vi "Get StartStop Status.vi"(8 "error in":errorcluster, 11 "VISA resource name in":refnum<visa-resource-name>) -> (0 "error out":errorcluster, 1 "Status":bool, 3 "VISA resource name out":refnum<visa-resource-name>)   [LabVIEW 2015, in "JULABO DeviceDriver.lvlib"]
doc: "This VI returns true if the instrument is started or false if it is in Standby-Mode"
uses:
  JULABO DeviceDriver.lvlib
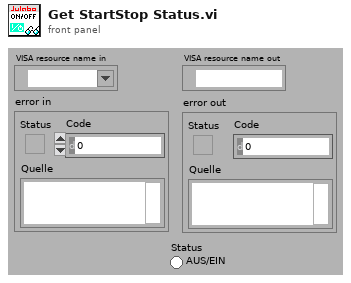
[diagram p1: front panel]
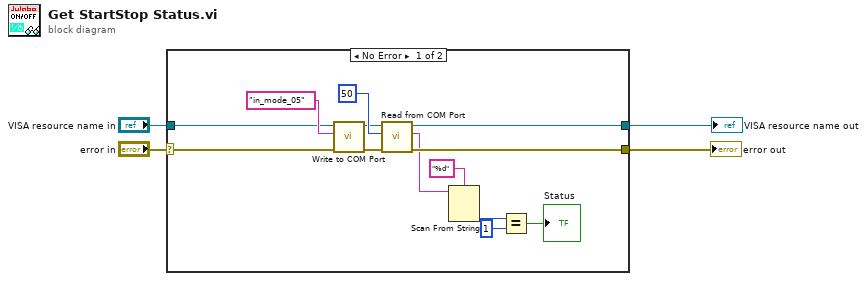
[diagram p0: block diagram]
diagram:
  n1 = case shown="No Error" "error in" {
    selector: "error in" -> [w5 w18]
    tunnel: [w16 w18] -> w4
    tunnel: [w13 w19] -> w3
    tunnel: "VISA resource name in" -> [w9 w19]
    frame No Error {
      n2 = call "Write to COM Port.vi"("error in"=w5, "Command (input)"="in_mode_05", "VISA resource name in"=w9) -> ("error out"=w10:errorcluster, "VISA resource name out"=w11:refnum<visa-resource-name>)  [unwired: 7 in]
      n3 = call "Read from COM Port.vi"("error in"=w10, "Byte to Read (-1:All)"=u32 50 ("Anzahl der Byte"), "VISA resource name in"=w11) -> ("error out"=w16:errorcluster, "String (output)"=w14:string, "VISA resource name out"=w13:refnum<visa-resource-name>)  [unwired: 5 in, 1 out]
      n4 = Scan From String(format string="%d" ("Format-String"), input string=w14) -> (output 1=w8:i32)  [unwired: 3 in, 3 out]
      n5 = Equal?(x=w8, y=1) -> (x = y?=→"Status":bool)
    }
    frame Error {
    }
  }
  "error out" <- w4
  "VISA resource name out" <- w3
